vi "Get Idents.vi"(11 "Buffer Lossless Digital in":refnum<class "Buffer Lossless Digital.lvclass">) -> (2 "Idents":string[](array[string]), 3 "Buffer Lossless Digital out":refnum<class "Buffer Lossless Digital.lvclass">)   [LabVIEW 2024, in "Buffer Lossless Digital.lvclass"]
uses:
  Buffer Lossless Digital.lvclass
  Buffer Lossless Digital.lvclass/Buffer Lossless Digital.ctl
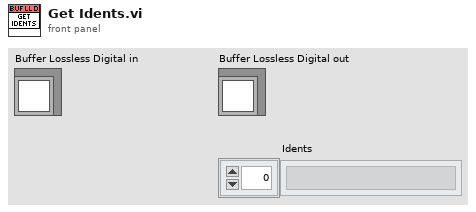
[diagram p1: front panel]
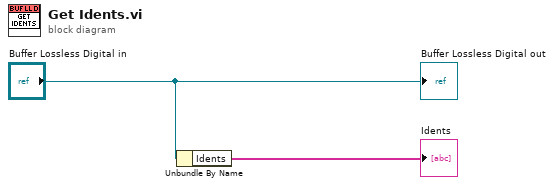
[diagram p0: block diagram]
diagram:
  n1 = Unbundle By Name("Buffer Lossless Digital in") -> ("Idents"=→"Idents":string[])
  "Buffer Lossless Digital out" <- "Buffer Lossless Digital in"
